vi "Temp_Calc.vi"(5 "aDATA":u8[](array[numeric])) -> (0 "Temp CH 1-4":dbl format="%#_3f", 1 "CPU Temp":dbl, 2 "Temp CH 5-9":dbl, 3 "Temp CH10 14":dbl, 4 "Temp CH 15 19":dbl)   [LabVIEW 2017]
uses:
  <vilib>/Analysis/NI_AALPro.lvlib
panel:
  out "RT (Ohms) 4":dbl
  out "RT (Ohms) 3":dbl
  out "RT (Ohms) 2":dbl
  out "RT (Ohms)":dbl
  out "RT":dbl[](array[numeric]) format="%0.2f"
  out "Temp":dbl[](array[numeric]) format="%0.2f"
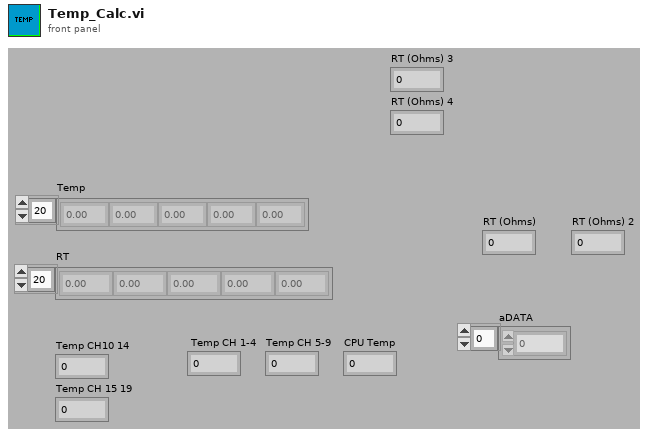
[diagram p1: front panel]
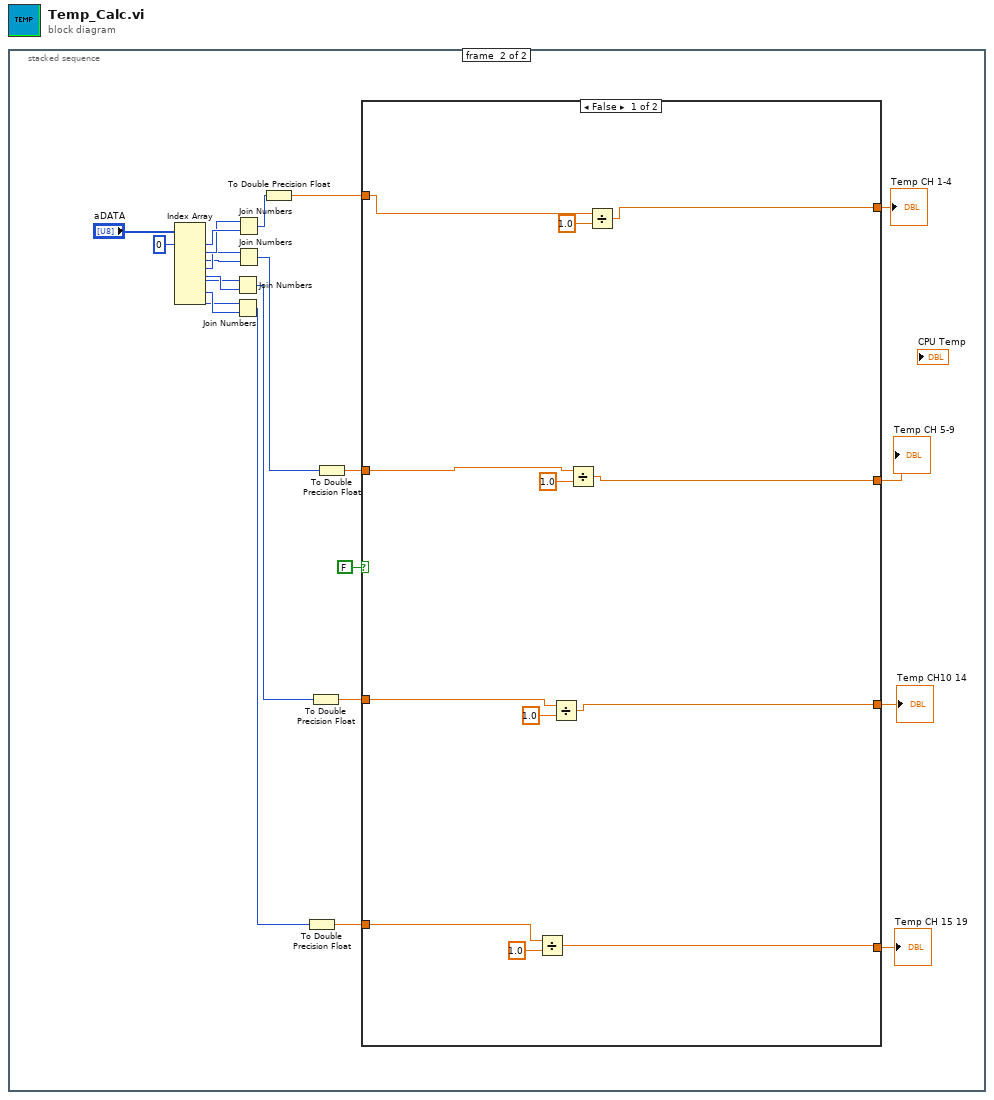
[diagram p0: block diagram]
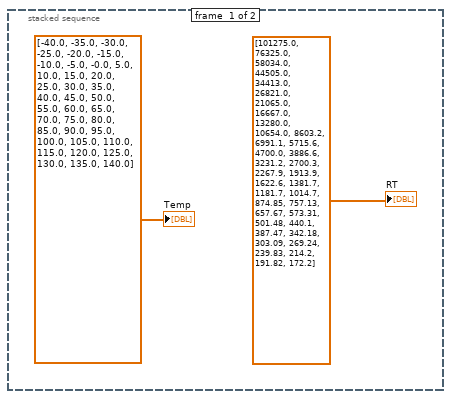
[diagram p2: hidden frame]
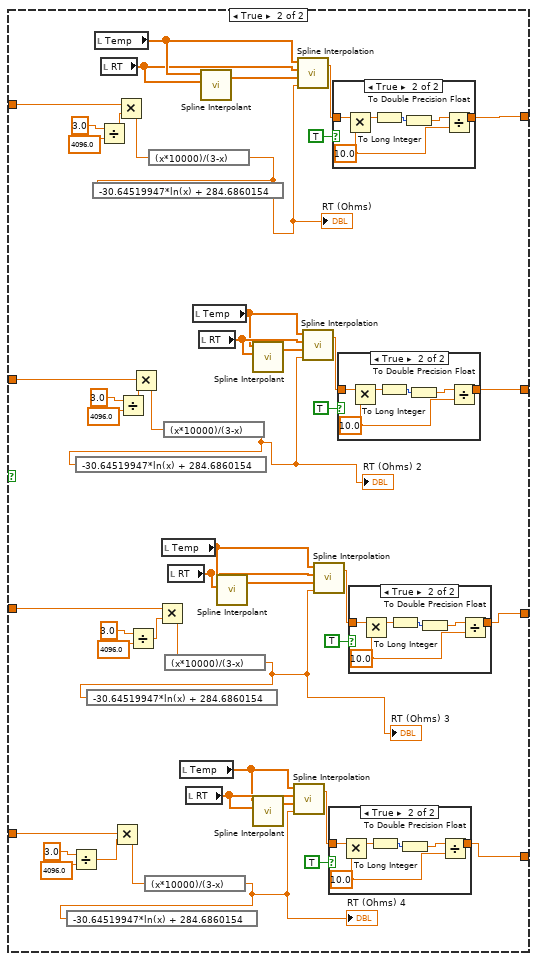
[diagram p3: hidden frame]
diagram:
  n1 = stacked-sequence {
    frame #0 {
      "Temp" <- dbl[] [-40.0, -35.0, -30.0, -25.0, -20.0, -15.0, -10.0, -5.0, -0.0, 5.0, 10.0, 15.0, 20.0, 25.0, 30.0, 35.0, 40.0, 45.0, 50.0, 55.0, 60.0, 65.0, 70.0, 75.0, 80.0, 85.0, 90.0, 95.0, 100.0, 105.0, 110.0, 115.0, 120.0, 125.0, 130.0, 135.0, 140.0] ("Temp")
      "RT" <- dbl[] [101275.0, 76325.0, 58034.0, 44505.0, 34413.0, 26821.0, 21065.0, 16667.0, 13280.0, 10654.0, 8603.2, 6991.1, 5715.6, 4700.0, 3886.6, 3231.2, 2700.3, 2267.9, 1913.9, 1622.6, 1381.7, 1181.7, 1014.7, 874.85, 757.13, 657.67, 573.31, 501.48, 440.1, 387.47, 342.18, 303.09, 269.24, 239.83, 214.2, 191.82, 172.2] ("RT")
    }
    frame #1 {
      n2 = Index Array(array="aDATA", index #1=0 ("index")) -> (element #1=w22:u8, element #2=w21:u8, element #3=w19:u8, element #4=w20:u8, element #5=w16:u8, element #6=w15:u8, element #7=w14:u8, element #8=w13:u8)  [unwired: 7 in]
      n3 = Join Numbers(hi=w15, lo=w16) -> ((hi.lo)=w5:u16)
      n4 = Join Numbers(hi=w13, lo=w14) -> ((hi.lo)=w4:u16)
      n5 = Join Numbers(hi=w21, lo=w22) -> ((hi.lo)=w24:u16)
      n6 = Join Numbers(hi=w20, lo=w19) -> ((hi.lo)=w6:u16)
      n7 = To Double Precision Float(number=w24) -> (double precision float=w25:dbl)
      n8 = To Double Precision Float(number=w4) -> (double precision float=w10:dbl)
      n9 = To Double Precision Float(number=w5) -> (double precision float=w11:dbl)
      n10 = To Double Precision Float(number=w6) -> (double precision float=w12:dbl)
      n11 = case shown="False" FALSE {
        tunnel: w25 -> [w37 w81]
        tunnel: [w36 w75] -> w17
        tunnel: w12 -> [w31 w67]
        tunnel: w11 -> [w29 w60]
        tunnel: w10 -> [w27 w48]
        tunnel: [w30 w44] -> w9
        tunnel: [w28 w43] -> w8
        tunnel: [w26 w42] -> w7
        frame False {
          n12 = Divide(x=w27, y=1.0) -> (x/y=w26:dbl)
          n13 = Divide(x=w29, y=1.0) -> (x/y=w28:dbl)
          n14 = Divide(x=w31, y=1.0) -> (x/y=w30:dbl)
          n15 = Divide(x=w37, y=1.0) -> (x/y=w36:dbl)
        }
        frame True {
          n16 = Divide(x=3.0, y=4096.0) -> (x/y=w38:dbl)
          n17 = local read "Temp"() -> (w85:dbl[])
          n18 = Divide(x=3.0, y=4096.0) -> (x/y=w76:dbl)
          n19 = local read "RT"() -> (w84:dbl[])
          n20 = Multiply(x=w48, y=w38) -> (x*y=w50:dbl)
          n21 = Multiply(x=w81, y=w76) -> (x*y=w79:dbl)
          n22 = Divide(x=3.0, y=4096.0) -> (x/y=w72:dbl)
          n23 = Divide(x=3.0, y=4096.0) -> (x/y=w55:dbl)
          n24 = Multiply(x=w67, y=w72) -> (x*y=w69:dbl)
          n25 = expression code="(x*10000)/(3-x)"(w50) -> (w39:dbl)
          "RT (Ohms) 4" <- w39
          n26 = expression code="-30.64519947*ln(x) + 284.6860154"(w39) -> ()  [unwired: 1 out]
          n27 = expression code="(x*10000)/(3-x)"(w79) -> (w82:dbl)
          "RT (Ohms)" <- w82
          n28 = expression code="-30.64519947*ln(x) + 284.6860154"(w82) -> ()  [unwired: 1 out]
          n29 = Multiply(x=w60, y=w55) -> (x*y=w58:dbl)
          n30 = local read "Temp"() -> (w63:dbl[])
          n31 = expression code="(x*10000)/(3-x)"(w69) -> (w41:dbl)
          "RT (Ohms) 2" <- w41
          n32 = expression code="-30.64519947*ln(x) + 284.6860154"(w41) -> ()  [unwired: 1 out]
          n33 = expression code="(x*10000)/(3-x)"(w58) -> (w40:dbl)
          "RT (Ohms) 3" <- w40
          n34 = expression code="-30.64519947*ln(x) + 284.6860154"(w40) -> ()  [unwired: 1 out]
          n35 = local read "RT"() -> (w62:dbl[])
          n36 = local read "Temp"() -> (w45:dbl[])
          n37 = local read "RT"() -> (w46:dbl[])
          n38 = local read "Temp"() -> (w64:dbl[])
          n39 = local read "RT"() -> (w65:dbl[])
          n40 = call <vilib>:"Spline Interpolant.vi"("X"=w84, "Y"=w85) -> ("Interpolant"=w80:dbl[])  [unwired: 2 in, 1 out]
          n41 = call <vilib>:"Spline Interpolant.vi"("X"=w62, "Y"=w63) -> ("Interpolant"=w59:dbl[])  [unwired: 2 in, 1 out]
          n42 = call <vilib>:"Spline Interpolant.vi"("X"=w65, "Y"=w64) -> ("Interpolant"=w68:dbl[])  [unwired: 2 in, 1 out]
          n43 = call <vilib>:"Spline Interpolant.vi"("X"=w46, "Y"=w45) -> ("Interpolant"=w49:dbl[])  [unwired: 2 in, 1 out]
          n44 = call <vilib>:"Spline Interpolation.vi"("x value"=w39, "Interpolant"=w49, "X"=w46, "Y"=w45) -> ("interpolation value"=w47:dbl)  [unwired: 1 out]
          n45 = call <vilib>:"Spline Interpolation.vi"("x value"=w82, "Interpolant"=w80, "X"=w84, "Y"=w85) -> ("interpolation value"=w83:dbl)  [unwired: 1 out]
          n46 = call <vilib>:"Spline Interpolation.vi"("x value"=w41, "Interpolant"=w68, "X"=w65, "Y"=w64) -> ("interpolation value"=w66:dbl)  [unwired: 1 out]
          n47 = call <vilib>:"Spline Interpolation.vi"("x value"=w40, "Interpolant"=w59, "X"=w62, "Y"=w63) -> ("interpolation value"=w61:dbl)  [unwired: 1 out]
          n48 = case shown="True" TRUE {
            tunnel: w47 -> [w86 w92]
            tunnel: [w86 w88] -> w42
            frame False {
            }
            frame True {
              w87 = 10.0 ("y")
              n49 = Multiply(x=w92, y=w87) -> (x*y=w91:dbl)
              n50 = To Long Integer(number=w91) -> (32bit integer=w90:i32)
              n51 = To Double Precision Float(number=w90) -> (double precision float=w89:dbl)
              n52 = Divide(x=w89, y=w87) -> (x/y=w88:dbl)
            }
          }
          n53 = case shown="True" TRUE {
            tunnel: w83 -> [w107 w113]
            tunnel: [w107 w109] -> w75
            frame False {
            }
            frame True {
              w108 = 10.0 ("y")
              n54 = Multiply(x=w113, y=w108) -> (x*y=w112:dbl)
              n55 = To Long Integer(number=w112) -> (32bit integer=w111:i32)
              n56 = To Double Precision Float(number=w111) -> (double precision float=w110:dbl)
              n57 = Divide(x=w110, y=w108) -> (x/y=w109:dbl)
            }
          }
          n58 = case shown="True" TRUE {
            tunnel: w66 -> [w100 w106]
            tunnel: [w100 w102] -> w44
            frame False {
            }
            frame True {
              w101 = 10.0 ("y")
              n59 = Multiply(x=w106, y=w101) -> (x*y=w105:dbl)
              n60 = To Long Integer(number=w105) -> (32bit integer=w104:i32)
              n61 = To Double Precision Float(number=w104) -> (double precision float=w103:dbl)
              n62 = Divide(x=w103, y=w101) -> (x/y=w102:dbl)
            }
          }
          n63 = case shown="True" TRUE {
            tunnel: w61 -> [w93 w99]
            tunnel: [w93 w95] -> w43
            frame False {
            }
            frame True {
              w94 = 10.0 ("y")
              n64 = Multiply(x=w99, y=w94) -> (x*y=w98:dbl)
              n65 = To Long Integer(number=w98) -> (32bit integer=w97:i32)
              n66 = To Double Precision Float(number=w97) -> (double precision float=w96:dbl)
              n67 = Divide(x=w96, y=w94) -> (x/y=w95:dbl)
            }
          }
        }
      }
      "Temp CH 1-4" <- w17
      "Temp CH 5-9" <- w9
      "Temp CH10 14" <- w8
      "Temp CH 15 19" <- w7
    }
  }
